vi "Set Voltage.vi"(7 "Position":u32, 8 "error in (no error)":errorcluster, 9 "Voltage Type":string, 10 "Voltage":dbl format="%#_13g", 11 "Driver Test in":refnum<class "Driver Test.lvclass">) -> (0 "error out":errorcluster)   [LabVIEW 2015, in "Driver Test.lvclass"]
doc: "Set voltage using recipe driven voltage type."
uses:
  Driver Test.lvclass
  CBTF Applications/Driver Board Testing/Main/Application/Application/Class/typedefs/Instrument Selector -- Enum.ctl
  Classes/Instruments/Power Supply/Class/Power Supply.lvclass
  Test Class/Test Class.lvclass
  CBTF Applications/Driver Board Testing/Main/Application/Application/Class/Driver Board Test.lvclass
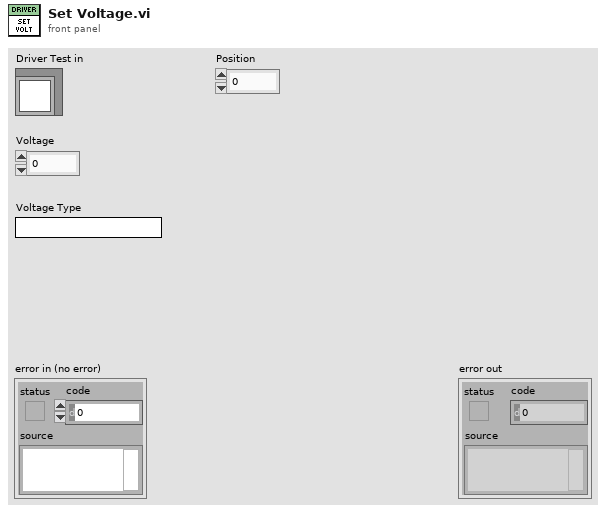
[diagram p1: front panel]
types:
  T1 = typedef "Driver Board Test.lvlib/Driver Board Test.lvclass/Instrument Selector -- Enum.ctl" = enum16{"ACPS1", "ACPS2", "DCPS1", "DCPS2", "DCPS3", "DCLoad1", "DCLoad2", "DPM1", "DPM2", "Switch1", "PXI1Slot2", "PXI1Slot3", "cDAQ1Mod5", "cDAQ1Mod6", "cDAQ1Mod7", "cDAQ1Mod8", "cDAQ1Mod1", "cDAQ1Mod2", "cDAQ1Mod3", "cDAQ1Mod4", "cDAQ2Mod1", "cDAQ2Mod2", "cDAQ2Mod3", "cDAQ2Mod4"}
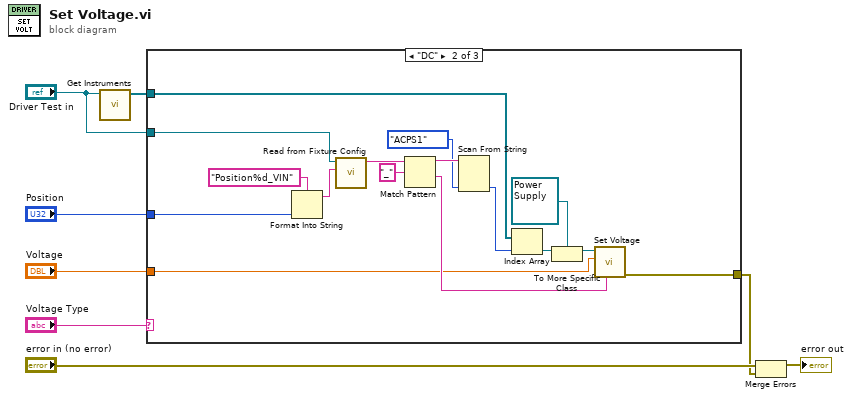
[diagram p0: block diagram]
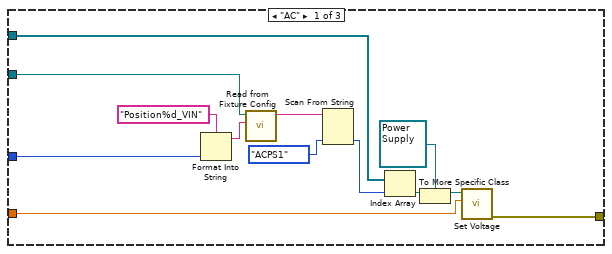
[diagram p2: hidden frame]
diagram:
  n1 = call "Get Instruments.vi"("Test Class in"="Driver Test in") -> ("Instruments"=w1:refnum<class "Instrument.lvclass">[])  [unwired: 9 in, 1 out]
  n2 = case shown="\"DC\"" "Voltage Type" {
    tunnel: "Voltage" -> [w11 w28 _]
    tunnel: [w10 w22 _] -> w2
    tunnel: "Position" -> [w13 w27 _]
    tunnel: "Driver Test in" -> [w14 w25 _]
    tunnel: w1 -> [w12 w23 _]
    frame "AC" {
      n3 = Format Into String(format string="Position%d_VIN", w13) -> (resulting string=w15:string)  [unwired: 2 in, 1 out]
      n4 = call-dynamic "Read from Fixture Config.vi"("Key"=w15, "Test Class in"=w14) -> ("Instrument Info"=w16:string)  [unwired: 8 in, 1 out]
      n5 = Scan From String(input string=w16, default 1=Instrument_Selector_--_Enum."ACPS1" ("Instrument")) -> (output 1=w19:T1)  [unwired: 3 in, 3 out]
      n6 = Index Array(array=w12, index=w19) -> (element=w20:refnum<class "Instrument.lvclass">)
      n7 = To More Specific Class(target class=refnum<class "Power Supply.lvclass"> refnum ("Power Supply.lvlib:Power Supply.lvclass"), reference=w20) -> (specific class reference=w21:refnum<class "Power Supply.lvclass">)  [unwired: 1 in, 1 out]
      n8 = call-dynamic "Set Voltage.vi"("Voltage (0.0 V)"=w11, "Acrobat Template in"=w21) -> ("error out"=w10:errorcluster)  [unwired: 8 in, 1 out]
    }
    frame "DC" {
      n9 = Format Into String(format string="Position%d_VIN", w27) -> (resulting string=w24:string)  [unwired: 2 in, 1 out]
      n10 = call-dynamic "Read from Fixture Config.vi"("Key"=w24, "Test Class in"=w25) -> ("Instrument Info"=w26:string)  [unwired: 8 in, 1 out]
      n11 = Match Pattern(string=w26, regular expression="_") -> (before substring=w36:string, after substring=w37:string)  [unwired: 1 in, 2 out]
      n12 = Scan From String(input string=w36, default 1=Instrument_Selector_--_Enum."ACPS1" ("Instrument")) -> (output 1=w31:T1)  [unwired: 3 in, 3 out]
      n13 = Index Array(array=w23, index=w31) -> (element=w32:refnum<class "Instrument.lvclass">)
      n14 = To More Specific Class(target class=refnum<class "Power Supply.lvclass"> refnum ("Power Supply.lvlib:Power Supply.lvclass"), reference=w32) -> (specific class reference=w33:refnum<class "Power Supply.lvclass">)  [unwired: 1 in, 1 out]
      n15 = call-dynamic "Set Voltage.vi"("Channel (\"1\")"=w37, "Voltage (0.0 V)"=w28, "Acrobat Template in"=w33) -> ("error out"=w22:errorcluster)  [unwired: 7 in, 1 out]
    }
    frame Default {
    }
  }
  n16 = Merge Errors("error in (no error)", w2) -> (→"error out":errorcluster)
